vi "conversion_ramp.vi"(7 "From Hz/ms to Driver":bool, 9 "Value":i32, 11 "Command":string) -> (1 "Value out":i32, 3 "String":string)   [LabVIEW 2013]
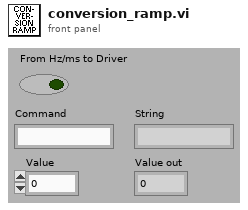
[diagram p1: front panel]
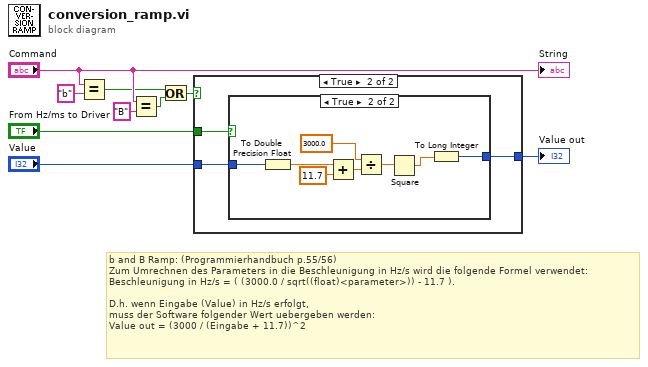
[diagram p0: block diagram]
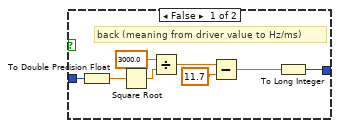
[diagram p3: hidden frame]
diagram:
  # "b and B Ramp: (Programmierhandbuch p.55/56)\nZum Umrechnen des Parameters in die Beschleunigung in Hz/s wird die folgende Formel verwendet:\nBeschleunigung in Hz/s = ( (3000.0 / sqrt((float)<parameter>)) - 11.7 ).\n\nD.h. wenn Eingabe (Value) in Hz/s erfolgt,\nmuss der Software folgender Wert uebergeben werden:\nValue out = (3000 / (Eingabe + 11.7))^2"
  n1 = Equal?(x="Command", y="b") -> (x = y?=w3:bool)
  n2 = Equal?(x="Command", y="B") -> (x = y?=w2:bool)
  n3 = Or(x=w3, y=w2) -> (x .or. y?=w1:bool)
  n4 = case shown="True" w1 {
    tunnel: "Value" -> [w10 w12]
    tunnel: [w10 w13] -> w7
    tunnel: "From Hz/ms to Driver" -> [_ w11]
    frame False {
    }
    frame True {
      n5 = case shown="True" w11 {
        tunnel: [w20 w29] -> w13
        tunnel: w12 -> [w19 w23]
        frame False {
          # "back (meaning from driver value to Hz/ms)"
          n6 = To Double Precision Float(number=w19) -> (double precision float=w17:dbl)
          n7 = Square Root(x=w17) -> (sqrt(x)=w21:dbl)
          n8 = Divide(x=3000.0, y=w21) -> (x/y=w16:dbl)
          n9 = Subtract(x=w16, y=11.7) -> (x-y=w14:dbl)
          n10 = To Long Integer(number=w14) -> (32bit integer=w20:i32)
        }
        frame True {
          n11 = To Double Precision Float(number=w23) -> (double precision float=w22:dbl)
          n12 = Add(x=w22, y=11.7) -> (x+y=w27:dbl)
          n13 = Divide(x=3000.0, y=w27) -> (x/y=w25:dbl)
          n14 = Square(x=w25) -> (x^2=w24:dbl)
          n15 = To Long Integer(number=w24) -> (32bit integer=w29:i32)
        }
      }
    }
  }
  "Value out" <- w7
  "String" <- "Command"
